vi "Probar y Calibrar Motores.vi"() -> ()   [LabVIEW 2013]
uses:
  <vilib>/Instr/_visa.llb/VISA Configure Serial Port (Instr).vi
panel:
  in  "Motor 4":u16(knob) scale=1000.0..2000.0
  in  "Motor 3":u16(knob) scale=1000.0..2000.0
  in  "Motor 2":u16(knob) scale=1000.0..2000.0
  in  "Motor 1":u16(knob) scale=1000.0..2000.0
  out "Datos enviados":string
  in  "stop":bool
  out "Datos recibidos":string
  in  "Puerto Serial":refnum<visa-resource-name>
  # "Probar y Calibrar Motores"
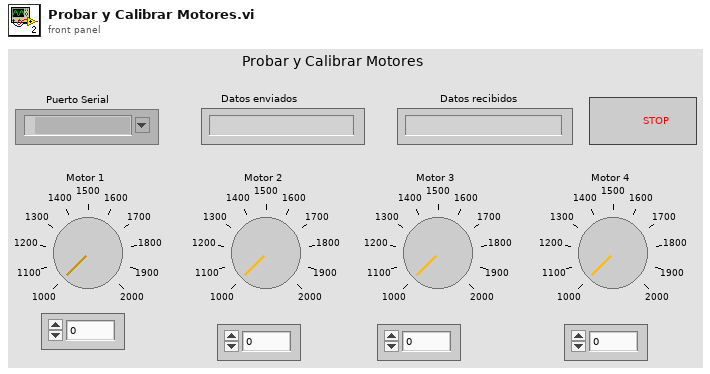
[diagram p1: front panel]
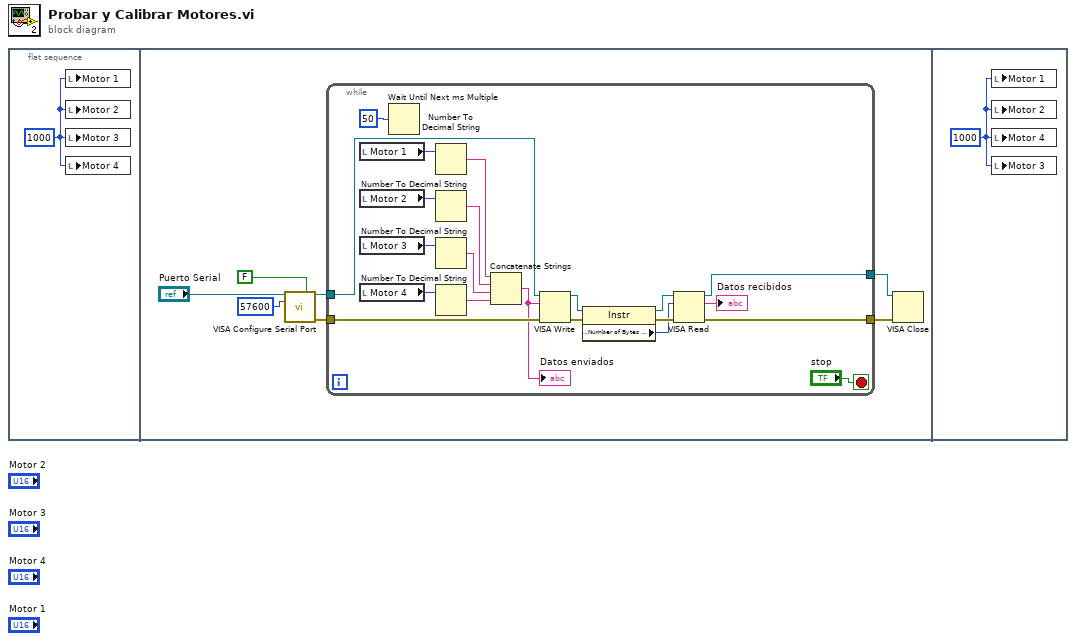
[diagram p0: block diagram]
diagram:
  n1 = flat-sequence {
    frame #0 {
      w1 = u16 1000 ("Pitch")
      n2 = local write "Motor 1"(w1) -> ()
      n3 = local write "Motor 2"(w1) -> ()
      n4 = local write "Motor 3"(w1) -> ()
      n5 = local write "Motor 4"(w1) -> ()
    }
    frame #1 {
      n6 = call-poly "VISA Configure Serial Port"("VISA resource name"="Puerto Serial", "Enable Termination\nChar (T)"=FALSE ("Enable Termination\nChar (T)"), "baud rate (9600)"=u32 57600) -> ("VISA resource name out"=w7:refnum<visa-resource-name>, "error out"=w5:errorcluster)  [unwired: 11 in]
      n7 = while {
        tunnel: w7 -> [w26]
        tunnel: [w24] -> w6
        tunnel: w5 -> [w23]
        tunnel: [w21] -> w4
        stop <- "stop" stop-if-true
        n8 = local read "Motor 1"() -> (w17:u16)
        n9 = local read "Motor 2"() -> (w16:u16)
        n10 = local read "Motor 3"() -> (w15:u16)
        n11 = local read "Motor 4"() -> (w14:u16)
        n12 = Wait Until Next ms Multiple(millisecond multiple=u32 50) -> ()  [unwired: 1 out]
        n13 = Number To Decimal String(number=w17) -> (decimal integer string=w13:string)  [unwired: 1 in]
        n14 = Number To Decimal String(number=w16) -> (decimal integer string=w12:string)  [unwired: 1 in]
        n15 = Number To Decimal String(number=w15) -> (decimal integer string=w11:string)  [unwired: 1 in]
        n16 = Number To Decimal String(number=w14) -> (decimal integer string=w10:string)  [unwired: 1 in]
        n17 = Concatenate Strings(w13, w12, w11, w10) -> (w9:string)
        "Datos enviados" <- w9
        n18 = VISA Write(VISA resource name=w26, write buffer=w9, error in (no error)=w23) -> (VISA resource name out=w25:refnum<visa-resource-name>, error out=w22:errorcluster)  [unwired: 1 out]
        n19 = property class="Instr"(reference=w25, error in=w22) -> (reference out=w27:refnum<visa-resource-name>, error out=w29:errorcluster, "Serial Settings:Number of Bytes at Serial Port"=w28:u32)
        n20 = VISA Read(VISA resource name=w27, byte count=w28, error in (no error)=w29) -> (VISA resource name out=w24:refnum<visa-resource-name>, read buffer=→"Datos recibidos":string, error out=w21:errorcluster)  [unwired: 1 out]
      }
      n21 = VISA Close(VISA resource name=w6, error in (no error)=w4) -> ()  [unwired: 1 out]
    }
    frame #2 {
      w30 = u16 1000 ("Pitch")
      n22 = local write "Motor 1"(w30) -> ()
      n23 = local write "Motor 2"(w30) -> ()
      n24 = local write "Motor 4"(w30) -> ()
      n25 = local write "Motor 3"(w30) -> ()
    }
  }
